vi "GetSerialNumber.vi"(7 "Timeout (ms)":u32=2000, 8 "Error In":errorcluster, 11 "Sierra M100 In":refnum<visa-resource-name>) -> (0 "Error Out":errorcluster, 2 "Serial Number":string, 3 "Sierra M100 Out":refnum<visa-resource-name>)   [LabVIEW 2012, in "Sierra-M100.lvlib"]
doc: "This VI get the serial number of the mass flow controller."
uses:
  Sierra-M100.lvlib
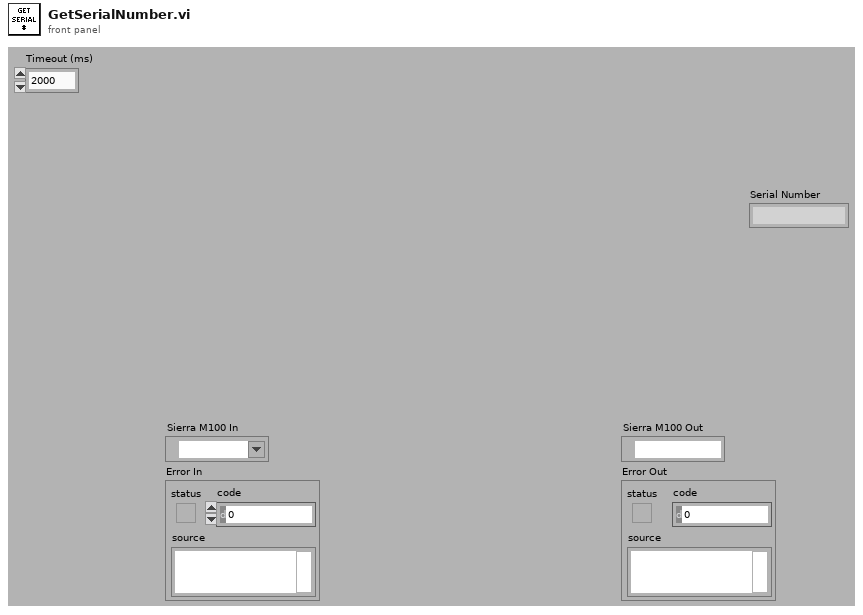
[diagram p1: front panel]
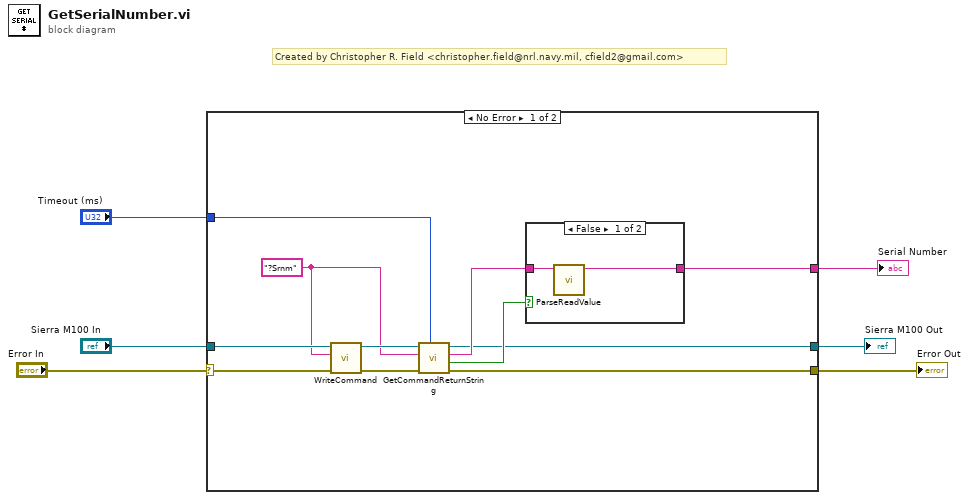
[diagram p0: block diagram]
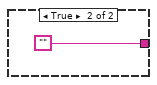
[diagram p2: hidden frame]
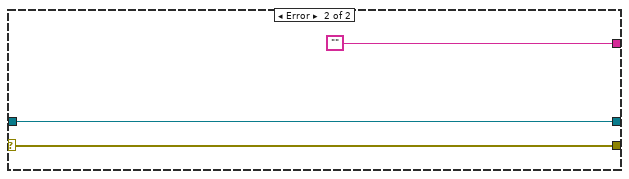
[diagram p3: hidden frame]
diagram:
  # "Created by Christopher R. Field <christopher.field@nrl.navy.mil, cfield2@gmail.com>"
  n1 = case shown="No Error" "Error In" {
    selector: "Error In" -> [w7 w22]
    tunnel: "Sierra M100 In" -> [w17 w23]
    tunnel: "Timeout (ms)" -> [w13 _]
    tunnel: [w10 ""] -> w4
    tunnel: [w9 w23] -> w3
    tunnel: [w8 w22] -> w2
    frame No Error {
      w14 = "?Srnm"
      n2 = call "WriteCommand.vi"("Error In"=w7, "Command"=w14, "Smart Trak 2 In"=w17) -> ("Error Out"=w15:errorcluster, "Smart Trak 2 Out"=w16:refnum<visa-resource-name>)  [unwired: 5 in, 2 out]
      n3 = call "GetCommandReturnString.vi"("Timeout (ms)"=w13, "Error In"=w15, "Command"=w14, "Smart Trak 2 In"=w16) -> ("Error Out"=w8:errorcluster, "Timeout?"=w12:bool, "Return String"=w11:string, "Smart Trak 2 Out"=w9:refnum<visa-resource-name>)  [unwired: 4 in]
      n4 = case shown="False" w12 {
        tunnel: w11 -> [w19 _]
        tunnel: [w18 ""] -> w10
        frame False {
          n5 = call "ParseReadValue.vi"("Read Buffer"=w19) -> ("Value"=w18:string)  [unwired: 10 in]
        }
        frame True {
        }
      }
    }
    frame Error {
    }
  }
  "Sierra M100 Out" <- w3
  "Error Out" <- w2
  "Serial Number" <- w4
